vi "Do.vi"(8 "error in (no error)":errorcluster, 10 "Actor in":refnum<class "Actor.lvclass">, 11 "Write Camera Settings Msg":refnum<class "Write Camera Settings Msg.lvclass">) -> (0 "error out":errorcluster, 2 "Actor out":refnum<class "Actor.lvclass">)   [LabVIEW 2014, in "HIJ IMAQdx Display.lvlib" / "Write Camera Settings Msg.lvclass"]
doc: "This VI delivers the message to the actor by calling the appropriate method(s) on the actor."
uses:
  Write Camera Settings Msg.lvclass
  <vilib>/ActorFramework/Actor/Actor.lvclass
  AF IMAQ Display/HIJ IMAQdx Display.lvclass
  Camera Actors/Camera Actor/Camera Actor Messages/Publish Camera Settings Msg/Publish Camera Settings Msg.lvclass
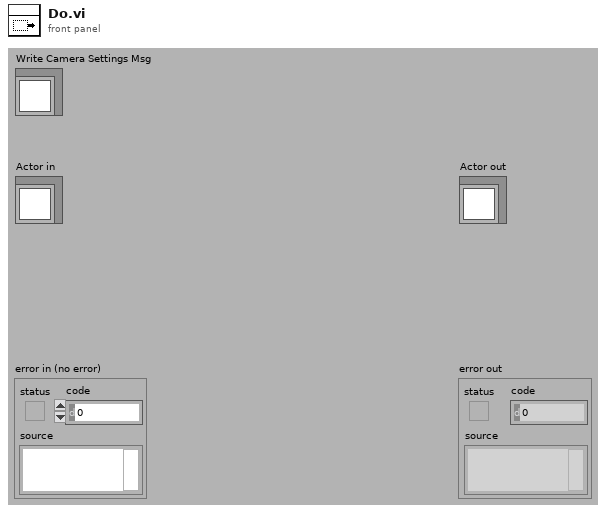
[diagram p1: front panel]
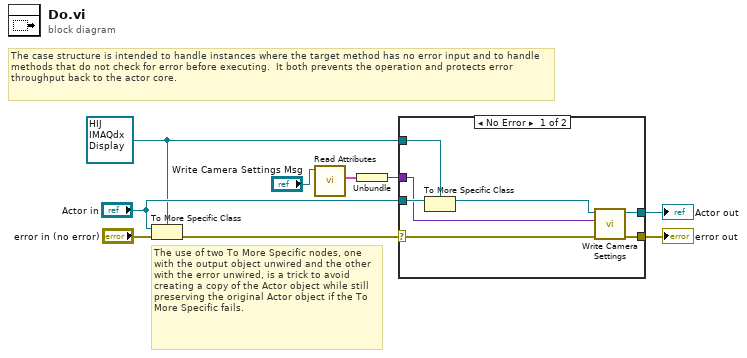
[diagram p0: block diagram]
diagram:
  w4 = refnum<class "HIJ IMAQdx Display.lvclass"> refnum ("Actor in")
  # "The use of two To More Specific nodes, one with the output object unwired and the other with the error unwired, is a trick to avoid creating a copy of the Actor object while still preserving the original Actor object if the To More Specific fails."
  # "The case structure is intended to handle instances where the target method has no error input and to handle methods that do not check for error before executing.  It both prevents the operation and protects error throughput back to the actor core."
  n1 = To More Specific Class(target class=w4, reference="Actor in", error in="error in (no error)") -> (error out=w8:errorcluster)  [unwired: 1 out]
  n2 = call "Read Attributes.vi"("Abstract Message Template in"="Write Camera Settings Msg") -> ("Payload"=w2:cluster{"Camera Settings":variant})  [unwired: 9 in, 1 out]
  n3 = Unbundle(w2) -> ("Camera Settings"=w1:variant)
  n4 = case shown="No Error" w8 {
    selector: w8 -> [w14 w18]
    tunnel: [w16 w18] -> w7
    tunnel: [w15 w17] -> w6
    tunnel: "Actor in" -> [w13 w17]
    tunnel: w4 -> [w12 _]
    tunnel: w1 -> [w11 _]
    frame No Error {
      n5 = To More Specific Class(target class=w12, reference=w13) -> (specific class reference=w10:refnum<class "HIJ IMAQdx Display.lvclass">)  [unwired: 1 in, 1 out]
      n6 = call-dynamic "Write Camera Settings.vi"("error in (no error)"=w14, "Camera Settings"=w11, "HIJ IMAQdx Display in"=w10) -> ("error out"=w16:errorcluster, "HIJ IMAQdx Display out"=w15:refnum<class "HIJ IMAQdx Display.lvclass">)  [unwired: 7 in]
    }
    frame Error {
      # "If type check fails, pass the original object out again."
    }
  }
  "error out" <- w7
  "Actor out" <- w6
